vi "find_peaks.vi"(6 "order":i32=4, 8 "freq":dbl=0.4 format="%#_13g", 9 "derivativePeak":bool, 10 "ranges":T1(array[cluster])=[{"min"=0.0, "max"=1000.0, "Sensibilidade"=50.0}] caption="Faixas" {"Sensibilidade" min=0.0 max=100.0 format="%#_g %"; "max" min=0.0 format="%#_g Hz"; "min" min=0.0 format="%#_g Hz"}, 11 "data":cluster{"freqs":dbl[], "Array":dbl[]}[](array[cluster])) -> (0 "d2x":cluster{"freqs":dbl[], "Array":dbl[]}[](array[cluster]), 1 "dx":cluster{"freqs":dbl[], "Array":dbl[]}[](array[cluster]), 2 "freqs":dbl[][](array[numeric]), 3 "plots":cluster{"Array":dbl[], "Array":dbl[]}[](array[cluster]))   [LabVIEW 2018]
uses:
  <vilib>/Analysis/NI_AAL_SigProc.lvlib
  <vilib>/gmath/NI_Gmath.lvlib
  <vilib>/Analysis/NI_AALPro.lvlib
panel:
  out "#freqs":i32[](array[numeric])
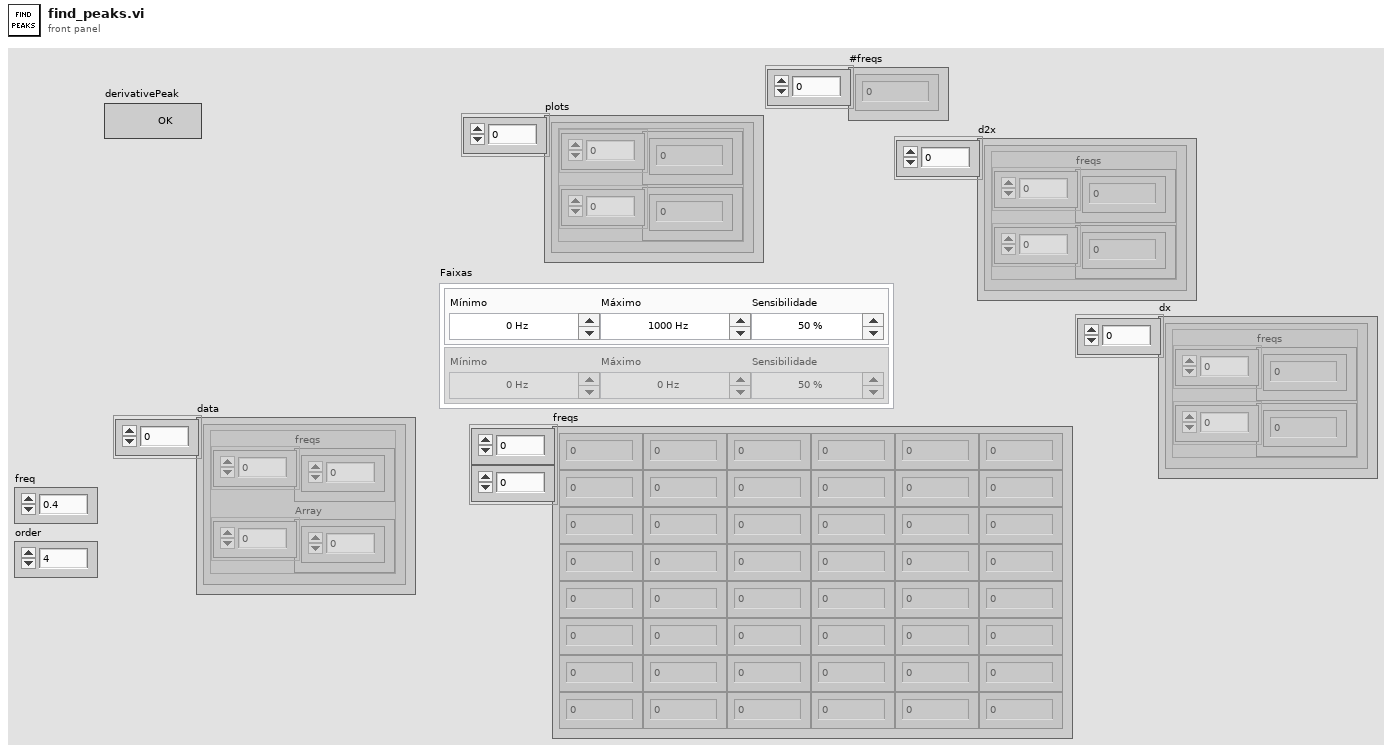
[diagram p1: front panel]
types:
  T1 = cluster{"min":dbl, "max":dbl, "Sensibilidade":dbl}[]
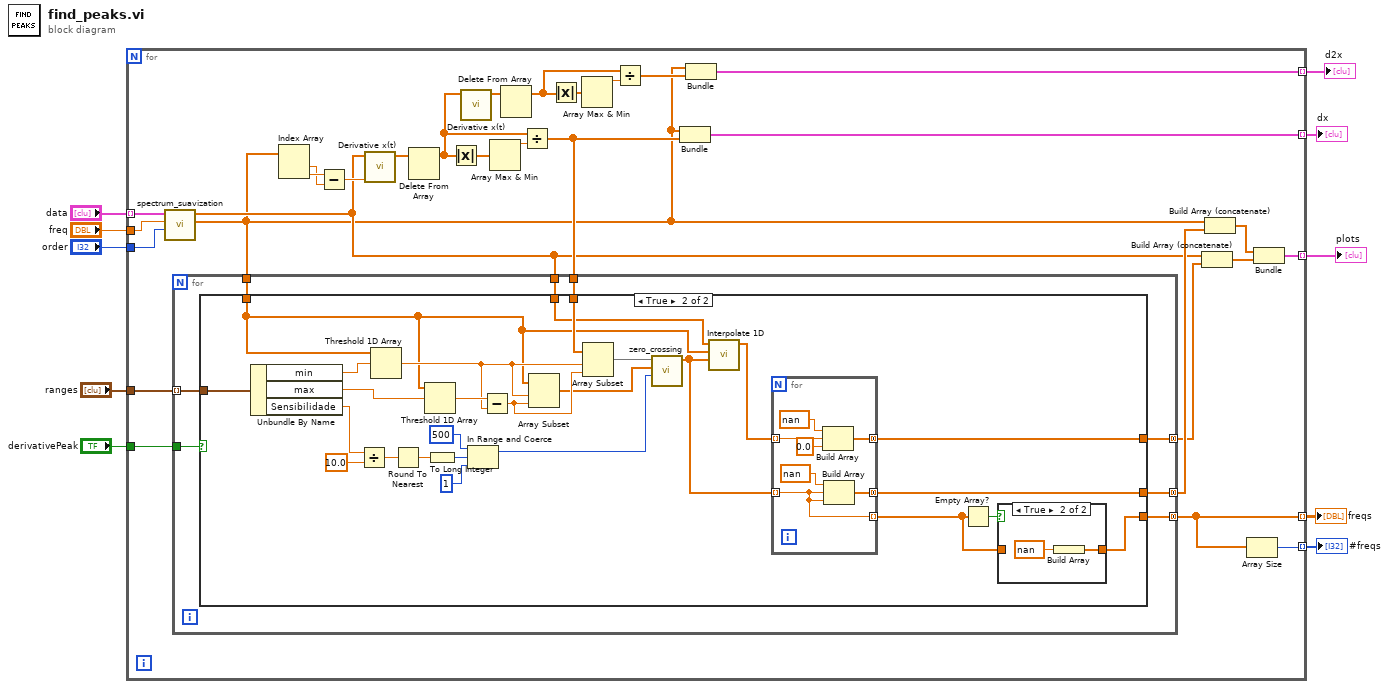
[diagram p0: block diagram]
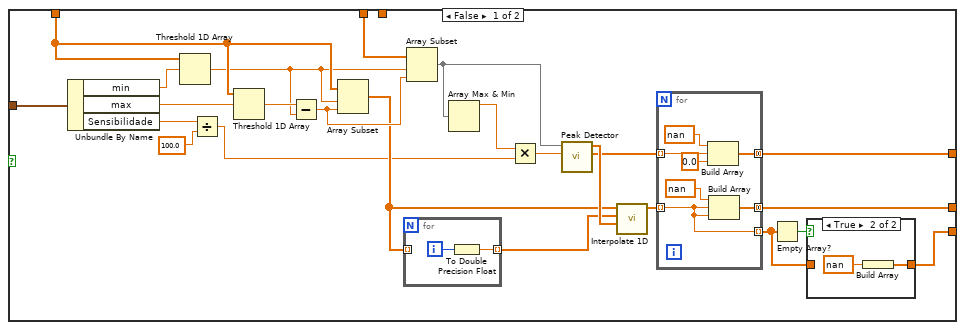
[diagram p2: hidden frame]
diagram:
  n1 = for {
    tunnel: "data" -> [w15] mode=indexing
    tunnel: "ranges" -> [w39]
    tunnel: [w16] -> w9 mode=indexing
    tunnel: [w34] -> w7 mode=indexing
    tunnel: [w33] -> w6 mode=indexing
    tunnel: [w24] -> w5 mode=indexing
    tunnel: [w23] -> w4 mode=indexing
    tunnel: "derivativePeak" -> [w18]
    tunnel: "freq" -> [w14]
    tunnel: "order" -> [w13]
    n2 = call "spectrum_suavization.vi"("order"=w13, "freq"=w14, "data"=w15) -> ("freqs"=w11:dbl[], "ampltiude"=w12:dbl[])  [unwired: 7 in]
    n3 = Index Array(array=w11) -> (element #1=w31:dbl, element #2=w32:dbl)  [unwired: 2 in]
    n4 = Subtract(x=w32, y=w31) -> (x-y=w30:dbl)
    n5 = call <vilib>:"Derivative x(t).vi"("dt"=w30, "X"=w12) -> ("dX/dt"=w22:dbl[])  [unwired: 8 in, 1 out]
    n6 = Delete From Array(array=w22) -> (array with subset deleted=w21:dbl[])  [unwired: 2 in, 1 out]
    n7 = Absolute Value(x=w21) -> (abs(x)=w29:dbl[])
    n8 = call <vilib>:"Derivative x(t).vi"("X"=w21) -> ("dX/dt"=w20:dbl[])  [unwired: 9 in, 1 out]
    n9 = Array Max & Min(array=w29) -> (max value=w28:dbl)  [unwired: 3 out]
    n10 = Delete From Array(array=w20) -> (array with subset deleted=w19:dbl[])  [unwired: 2 in, 1 out]
    n11 = Divide(x=w21, y=w28) -> (x/y=w17:dbl[])
    n12 = for {
      tunnel: w11 -> [w46]
      tunnel: w39 -> [w47] mode=indexing
      tunnel: [w45] -> w35 mode=concatenating
      tunnel: [w44] -> w36 mode=concatenating
      tunnel: [w43] -> w34 mode=concatenating
      tunnel: w18 -> [w42]
      tunnel: w17 -> [w41]
      tunnel: w12 -> [w40]
      n13 = case shown="True" w42 {
        tunnel: w47 -> [w71 w109]
        tunnel: w46 -> [w67 w94]
        tunnel: [w56 w103] -> w45
        tunnel: [w55 w102] -> w44
        tunnel: [w50 w100] -> w43
        tunnel: w41 -> [_ w98]
        tunnel: w40 -> [w48 w84]
        frame False {
          n14 = Unbundle By Name(w71) -> ("min"=w70:dbl, "max"=w69:dbl, "Sensibilidade"=w53:dbl)
          n15 = Threshold 1D Array(2:w70, 3:w67) -> (0:w66:dbl)  [unwired: 1 in]
          n16 = Divide(x=w53, y=100.0) -> (x/y=w52:dbl)
          n17 = Threshold 1D Array(2:w69, 3:w67) -> (0:w68:dbl)  [unwired: 1 in]
          n18 = Subtract(x=w68, y=w66) -> (x-y=w65:dbl)
          n19 = Array Subset(array=w67, index=w66, length=w65) -> (w60:dbl[])
          n20 = for {
            tunnel: w60 -> [_] mode=indexing
            tunnel: [w73] -> w59 mode=indexing
            i -> [w72]
            n21 = To Double Precision Float(number=w72) -> (double precision float=w73:dbl)
          }
          n22 = Array Subset(array=w48, index=w66, length=w65) -> (w62:dbl[])
          n23 = Array Max & Min(array=w62) -> (max value=w64:dbl)  [unwired: 3 out]
          n24 = Multiply(x=w64, y=w52) -> (x*y=w63:dbl)
          n25 = call <vilib>:"Peak Detector.vi"("threshold"=w63, "X"=w62) -> ("Amplitudes"=w57:dbl[], "Locations"=w61:dbl[])  [unwired: 5 in, 3 out]
          n26 = call <vilib>:"Interpolate 1D.vi"("xi"=w61, "X"=w59, "Y"=w60) -> ("yi"=w58:dbl[])  [unwired: 6 in, 2 out]
          n27 = for {
            tunnel: w58 -> [w77] mode=indexing
            tunnel: w57 -> [w83] mode=indexing
            tunnel: [w80] -> w55 mode=concatenating
            tunnel: [w79] -> w56 mode=concatenating
            tunnel: [w77] -> w49 mode=indexing
            n28 = Build Array(nan ("element"), w83, 0.0 ("element")) -> (w79:dbl[])
            n29 = Build Array(nan ("element"), w77, w77) -> (w80:dbl[])
          }
          n30 = Empty Array?(array=w49) -> (empty?=w51:bool)
          n31 = case shown="True" w51 {
            tunnel: [w74 w75] -> w50
            tunnel: w49 -> [w74 _]
            frame False {
            }
            frame True {
              n32 = Build Array(nan ("element")) -> (w75:dbl[])
            }
          }
        }
        frame True {
          n33 = Unbundle By Name(w109) -> ("min"=w108:dbl, "max"=w107:dbl, "Sensibilidade"=w92:dbl)
          n34 = Divide(x=w92, y=10.0) -> (x/y=w90:dbl)
          n35 = Threshold 1D Array(2:w108, 3:w94) -> (0:w105:dbl)  [unwired: 1 in]
          n36 = Round To Nearest(number=w90) -> (nearest integer value=w89:dbl)
          n37 = Threshold 1D Array(2:w107, 3:w94) -> (0:w106:dbl)  [unwired: 1 in]
          n38 = To Long Integer(number=w89) -> (32bit integer=w88:i32)
          n39 = In Range and Coerce(upper limit=500 ("lower limit"), x=w88, lower limit=1) -> (coerced(x)=w85:i32)  [unwired: 1 out]
          n40 = Subtract(x=w106, y=w105) -> (x-y=w104:dbl)
          n41 = Array Subset(array=w94, index=w105, length=w104) -> (w93:dbl[])
          n42 = Array Subset(array=w98, index=w105, length=w104) -> (w97:dbl[])
          n43 = call "zero_crossing.vi"("N"=w85, "freqs"=w93, "derivative"=w97) -> ("zero_pos"=w95:dbl[])  [unwired: 8 in]
          n44 = call <vilib>:"Interpolate 1D.vi"("xi"=w95, "X"=w94, "Y"=w84) -> ("yi"=w96:dbl[])  [unwired: 6 in, 2 out]
          n45 = for {
            tunnel: w95 -> [w113] mode=indexing
            tunnel: w96 -> [w119] mode=indexing
            tunnel: [w116] -> w102 mode=concatenating
            tunnel: [w115] -> w103 mode=concatenating
            tunnel: [w113] -> w99 mode=indexing
            n46 = Build Array(nan ("element"), w119, 0.0 ("element")) -> (w115:dbl[])
            n47 = Build Array(nan ("element"), w113, w113) -> (w116:dbl[])
          }
          n48 = Empty Array?(array=w99) -> (empty?=w101:bool)
          n49 = case shown="True" w101 {
            tunnel: [w110 w111] -> w100
            tunnel: w99 -> [w110 _]
            frame False {
            }
            frame True {
              n50 = Build Array(nan ("element")) -> (w111:dbl[])
            }
          }
        }
      }
    }
    n51 = Absolute Value(x=w19) -> (abs(x)=w26:dbl[])
    n52 = Array Max & Min(array=w26) -> (max value=w27:dbl)  [unwired: 3 out]
    n53 = Divide(x=w19, y=w27) -> (x/y=w25:dbl[])
    n54 = Bundle("freqs"=w11, w17) -> (w23:cluster{"freqs":dbl[], dbl[]})  [unwired: 1 in]
    n55 = Bundle("freqs"=w11, w25) -> (w24:cluster{"freqs":dbl[], dbl[]})  [unwired: 1 in]
    n56 = Build Array (concatenate)(w12, w35) -> (w37:dbl[])
    n57 = Build Array (concatenate)(w11, w36) -> (w38:dbl[])
    n58 = Array Size(array=w34) -> (size(s)=w33:i32)
    n59 = Bundle(w38, w37) -> (w16:cluster{dbl[], dbl[]})  [unwired: 1 in]
  }
  "plots" <- w9
  "freqs" <- w7
  "#freqs" <- w6
  "d2x" <- w5
  "dx" <- w4
